vi "Launch Chart.vi"   [LabVIEW 2020]
uses:
  modules/mva-viewable/Source/IViewModel/IViewModel/IViewModel.lvclass
  <vilib>/ActorFramework/Actor/Actor.lvclass
  modules/mva-core/Source/Mediator/Mediator/Mediator.lvclass
  modules/mva-viewable/Source/IViewable/IViewable Messages/Open Front Panel Msg/Open Front Panel Msg.lvclass
  <vilib>/ActorFramework/Message Enqueuer/Message Priority.ctl
  <vilib>/ActorFramework/Message Enqueuer/Message Enqueuer.lvclass
  modules/mva-viewable/Source/IViewable/IViewable/View Position Enum.ctl
  modules/mva-viewable/Source/IViewable/IViewable/IViewable.lvclass
  SimpleChart/SimpleChart.lvclass
  ExampleSimpleRootModel/SimpleRootModel.lvclass
  158084ce-0d1a-4c6f-81cb-d0b1039f64dd.vi
  C:/Program Files/National Instruments/LabVIEW 2020/vi.lib/ActorFramework/Actor/Actor.lvclass
panel:
  # "This example launches a simple chart MVA application"
types:
  T1 = typedef "MVA Framework.lvlib/IViewable.lvlib/IViewable.lvclass/View Position Enum.ctl" = enum16{"Centered", "Maximized", "Minimized", "Custom", "Unchanged"}
  T2 = typedef "Actor Framework.lvlib/Message Enqueuer.lvclass/Message Priority.ctl" = enum16{"Low", "Normal", "High"}
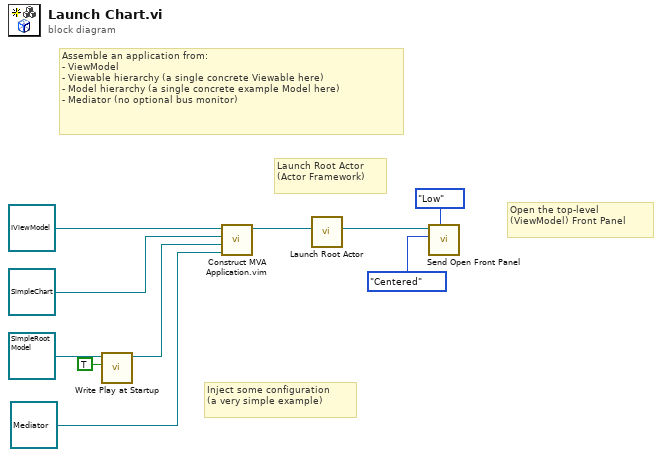
[diagram p0: block diagram]
diagram:
  # "Inject some configuration\n(a very simple example)"
  # "Open the top-level\n(ViewModel) Front Panel"
  # "Launch Root Actor\n(Actor Framework)"
  # "Assemble an application from:\n- ViewModel\n- Viewable hierarchy (a single concrete Viewable here)\n- Model hierarchy (a single concrete example Model here)\n- Mediator (no optional bus monitor)"
  n1 = call "Write Play at Startup.vi"("Play at Startup?"=TRUE, "SimpleRootModel in"=refnum<class "SimpleRootModel.lvclass"> refnum ("MVAExamples.lvlib:SimpleRootModel.lvclass")) -> ("SimpleRootModel out"=w3:refnum<class "SimpleRootModel.lvclass">)  [unwired: 9 in]
  n2 = call "Construct MVA Application.vim"("Mediator Type"=refnum<class "Mediator.lvclass"> refnum ("Mediator.lvlib:Mediator.lvclass"), "Model Type"=w3, "Startup View Configuration"=refnum<class "SimpleChart.lvclass"> refnum ("MVAExamples.lvlib:SimpleChart.lvclass"), "IViewModel In"=refnum<class "IViewModel.lvclass"> refnum ("IViewModel.lvlib:IViewModel.lvclass")) -> ("IViewModel Out"=w7:refnum<class "IViewModel.lvclass">)  [unwired: 7 in]
  n3 = call <vilib>:"Launch Root Actor.vi"("Actor"=w7) -> ("Actor's Enqueuer"=w6:refnum<class "Message Enqueuer.lvclass">)  [unwired: 9 in, 1 out]
  n4 = call "Send Open Front Panel.vi"("Message Priority (Normal)"=Message_Priority."Low", "Position"=View_Position_Enum."Centered", "Message Enqueuer"=w6) -> ()  [unwired: 7 in, 2 out]
